vi "DMMs_measure.vi"(0 "DMMsData in":refnum<class "DMMsData.lvclass">, 1 "Sample #":i32=5, 5 "MeasurementIndex":i32, 9 "SourceDataLabels":string[][](array[string]), 11 "error in (no error)":errorcluster, 12 "SourceDataArray":dbl[][](array[numeric])) -> (3 "TimeArray":timestamp[](array[timestamp]), 4 "DMMsData out":refnum<class "DMMsData.lvclass">, 6 "LastData":dbl[](array[numeric]), 10 "DataArray":dbl[][](array[numeric]), 14 "DeviceActive?":bool[](array[boolean]), 15 "error out":errorcluster)   [LabVIEW 2017, in "DMMsData.lvclass"]
uses:
  DMMsData.lvclass
  DMMsData.lvclass/DMMsData.ctl
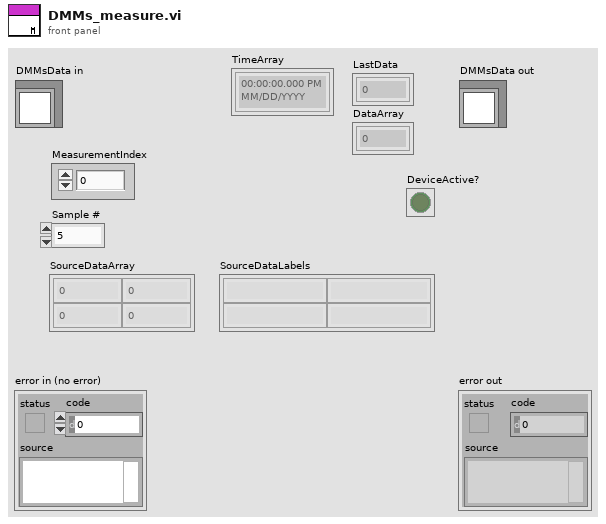
[diagram p1: front panel]
types:
  T1 = cluster{"Label":string, "Active?":bool, "Source":enum16{"USB6210", "USB6218AI", "USB6218AO", "LSI218", "LSI336"}, "SourceLabel":string, "FileFormat":string}[]
  T2 = cluster{"Label":string, "Active?":bool, "VISA resource name":refnum<visa-resource-name>, "Device":enum16{"Agilent34401A", "ADCMT7351", "HP3478A"}, "Measurement":enum16{"DC Volts", "DC Currents", "2-Wire Resistance", "4-Wire Resistance"}, "FileFormat":string}[]
  T3 = enum16{"DC Volts", "DC Currents", "2-Wire Resistance", "4-Wire Resistance"}
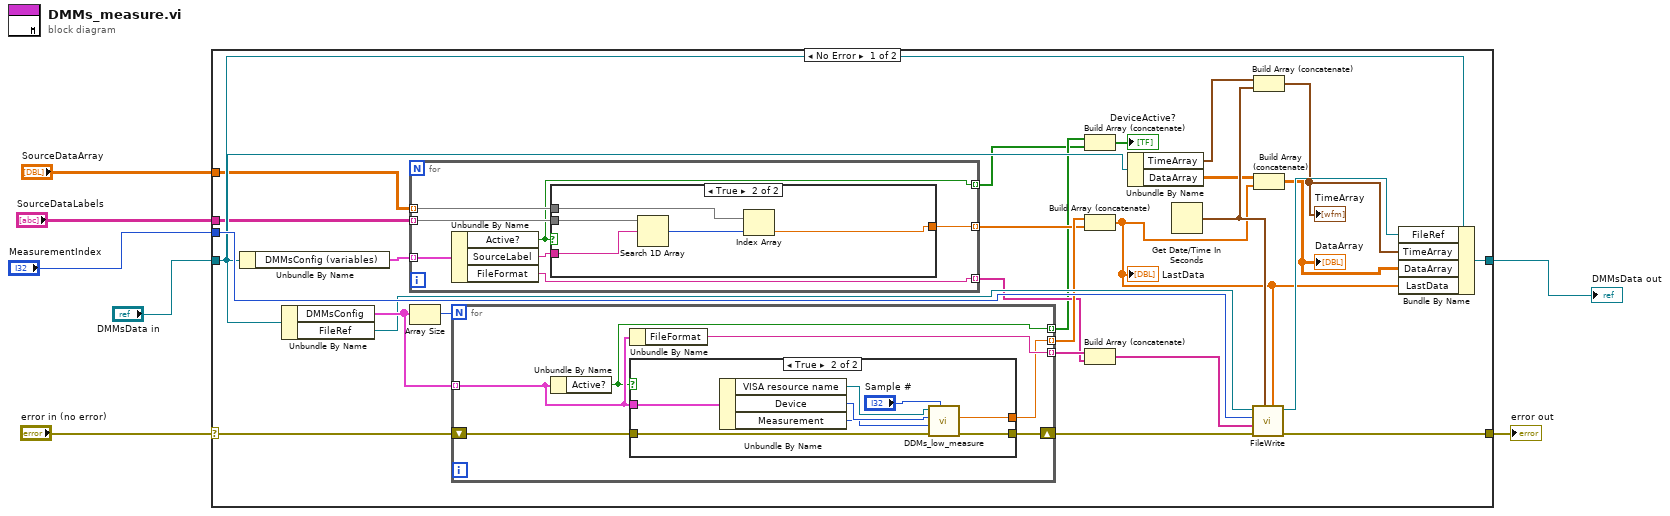
[diagram p0: block diagram]
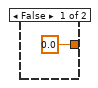
[diagram p2: hidden frame]
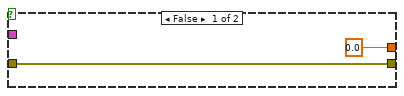
[diagram p3: hidden frame]
diagram:
  n1 = case shown="No Error" "error in (no error)" {
    selector: "error in (no error)" -> [w32 w65]
    tunnel: [w28 w65] -> w6
    tunnel: [w27 w64] -> w4
    tunnel: "DMMsData in" -> [w20 w64]
    tunnel: "MeasurementIndex" -> [w31 _]
    tunnel: "SourceDataArray" -> [w18 _]
    tunnel: "SourceDataLabels" -> [w17 _]
    frame No Error {
      n2 = Unbundle By Name(w20) -> ("DMMsConfig (variables)"=w19:T1)
      n3 = Unbundle By Name(w20) -> ("DMMsConfig"=w33:T2, "FileRef"=w30:refnum<file>)
      n4 = for {
        tunnel: w19 -> [w41] mode=indexing
        tunnel: w18 -> [w38] mode=indexing
        tunnel: w17 -> [w39] mode=indexing
        tunnel: [w37] -> w15 mode=indexing
        tunnel: [w36] -> w12 mode=indexing
        tunnel: [w35] -> w9 mode=indexing
        n5 = Unbundle By Name(w41) -> ("Active?"=w35:bool, "SourceLabel"=w40:string, "FileFormat"=w36:string)
        n6 = case shown="True" w35 {
          tunnel: w40 -> [_ w47]
          tunnel: w39 -> [_ w46]
          tunnel: w38 -> [_ w45]
          tunnel: [0.0 ("Numeric") w43] -> w37
          frame False {
          }
          frame True {
            n7 = Search 1D Array(1D array=w46, element=w47) -> (index of element=w44:i32)  [unwired: 1 in]
            n8 = Index Array(array=w45, index=w44) -> (element=w43:dbl)
          }
        }
      }
      n9 = Array Size(array=w33) -> (size(s)=w34:i32)
      n10 = for {
        N: w34 -> [_]
        tunnel: w33 -> [w53] mode=indexing
        shift-right: [w51] -> w29
        shift-left: w32 -> [w52]
        tunnel: [w50] -> w13 mode=indexing
        tunnel: [w49] -> w16 mode=indexing
        tunnel: [w48] -> w10 mode=indexing
        n11 = Unbundle By Name(w53) -> ("Active?"=w48:bool)
        n12 = Unbundle By Name(w53) -> ("FileFormat"=w50:string)
        n13 = case shown="True" w48 {
          tunnel: w53 -> [_ w63]
          tunnel: w52 -> [w55 w60]
          tunnel: [w55 w59] -> w51
          tunnel: [0.0 ("Measurement") w58] -> w49
          frame False {
          }
          frame True {
            n14 = Unbundle By Name(w63) -> ("VISA resource name"=w62:refnum<visa-resource-name>, "Device"=w61:enum16{"Agilent34401A", "ADCMT7351", "HP3478A"}, "Measurement"=w57:T3)
            n15 = call "DDMs_low_measure.vi"("Sample #"="Sample #", "error in (no error)"=w60, "Measurement"=w57, "Device"=w61, "VISA resource name"=w62) -> ("error out"=w59:errorcluster, "Measurement"=w58:dbl)  [unwired: 4 in, 1 out]
          }
        }
      }
      n16 = Build Array (concatenate)(w10, w9) -> (→"DeviceActive?":bool[])
      n17 = Build Array (concatenate)(w16, w15) -> (w14:dbl[])
      "LastData" <- w14
      n18 = Build Array (concatenate)(w13, w12) -> (w11:string[])
      n19 = Unbundle By Name(w20) -> ("TimeArray"=w25:timestamp[], "DataArray"=w22:dbl[][])
      n20 = Get Date/Time In Seconds() -> (seconds since 1Jan1904=w24:timestamp)
      n21 = call "FileWrite.vi"("DataArray"=w14, "Time Stamp"=w24, "Error In"=w29, "FileFormat"=w11, "Index"=w31, "refnum in"=w30) -> ("Error Out"=w28:errorcluster, "Byte Stream File Refnum"=w26:refnum<file>)  [unwired: 4 in]
      n22 = Build Array (concatenate)(w25, w24) -> (w23:timestamp[])
      "TimeArray" <- w23
      n23 = Build Array (concatenate)(w22, w14) -> (w21:dbl[][])
      "DataArray" <- w21
      n24 = Bundle By Name(cluster=w20, "FileRef"=w26, "TimeArray"=w23, "DataArray"=w21, "LastData"=w14) -> (w27:refnum<class "DMMsData.lvclass">)
    }
    frame Error {
    }
  }
  "error out" <- w6
  "DMMsData out" <- w4
